vi "2.1 Read Sensor Data.vi"() -> ()   [LabVIEW 2011]
uses:
  <vilib>/Instr/_visa.llb/VISA Configure Serial Port (Instr).vi
panel:
  out "concatenated string":string
  in  "Status":enum16{"Waiting", "Reading", "Time Out!"}(ring)
  in  "stop":bool
  out "Current Status":enum16{"Waiting", "Reading", "Time Out!"}(ring)
  in  "VISA resource name":refnum<visa-resource-name>="COM1"
  in  "error in (no error)":errorcluster
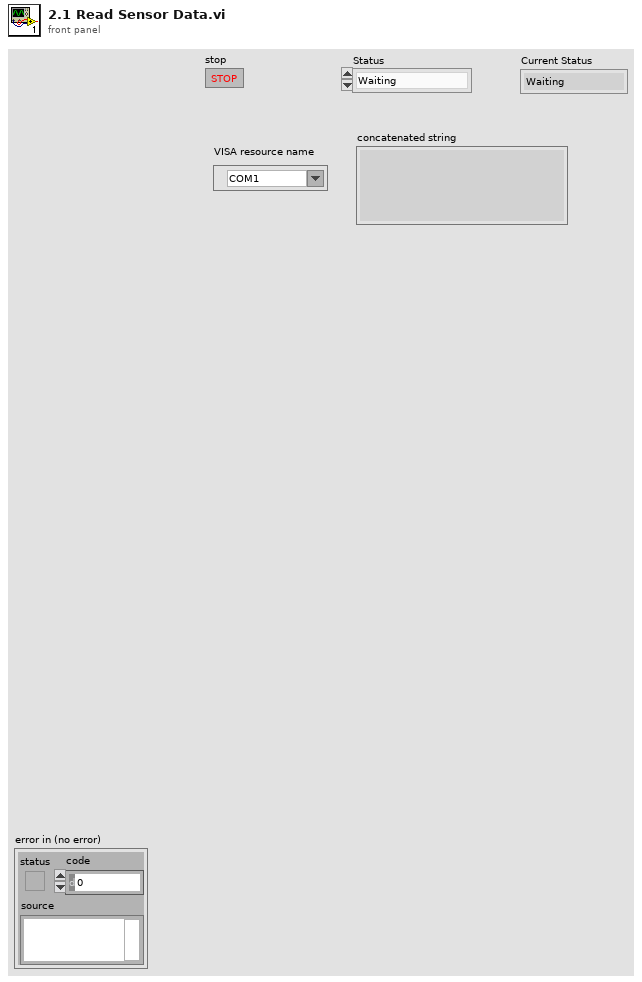
[diagram p1: front panel]
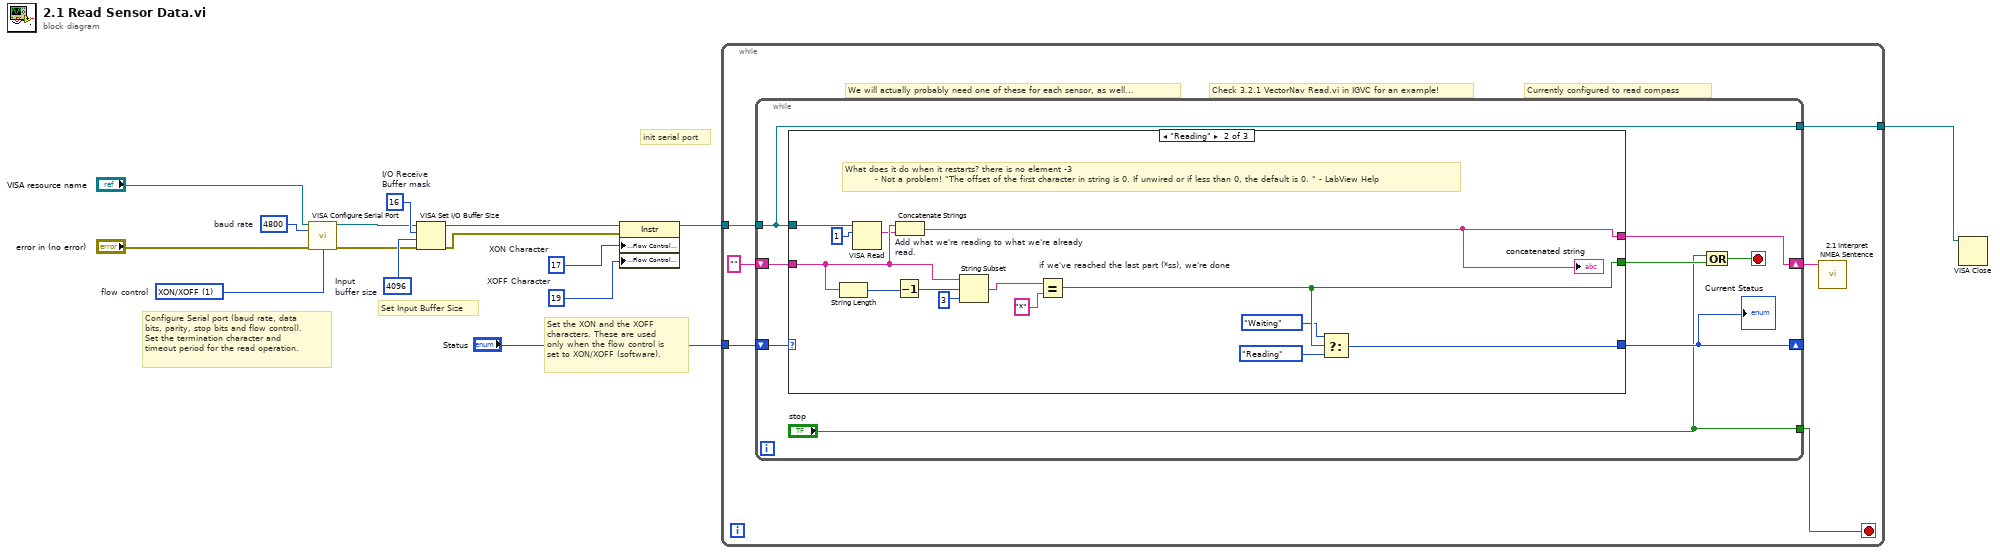
[diagram p0: block diagram]
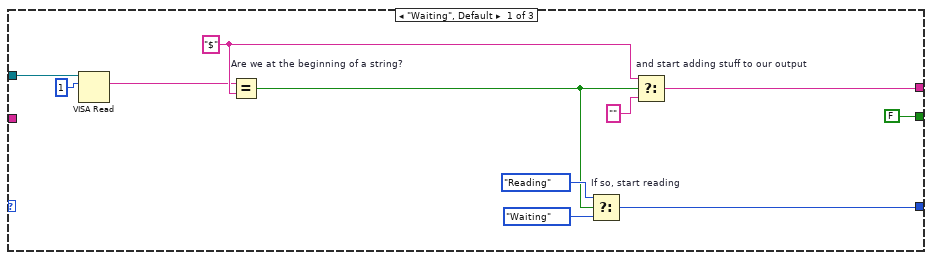
[diagram p2: hidden frame]
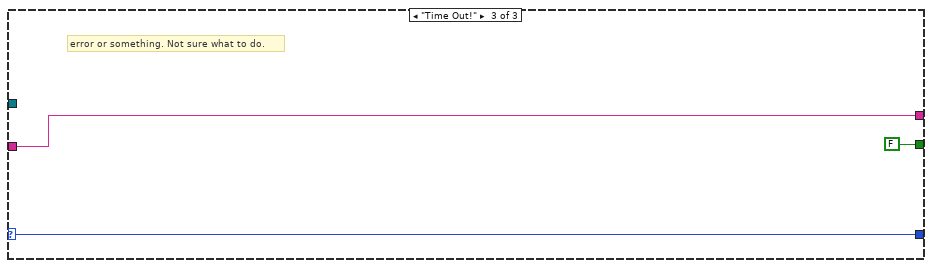
[diagram p3: hidden frame]
diagram:
  w5 = u8 19  # XOFF Character
  w6 = u8 17  # XON Character
  w9 = u32 4096  # Input buffer size
  w10 = u16 16  # I/O Receive Buffer mask
  w12 = u16 1 items=["None"=0, "XON/XOFF"=1, "RTS/CTS"=2, "DTR/DSR"=4]  # flow control
  w14 = u32 4800  # baud rate
  # "Set the XON and the XOFF\ncharacters. These are used\nonly when the flow control is\nset to XON/XOFF (software)."
  # "Set Input Buffer Size"
  # "init serial port"
  # "Configure Serial port (baud rate, data\nbits, parity, stop bits and flow control).\nSet the termination character and\ntimeout period for the read operation."
  n1 = call-poly "VISA Configure Serial Port"("VISA resource name"="VISA resource name", "baud rate (9600)"=w14, "error in (no error)"="error in (no error)", "flow control (0:none)"=w12) -> ("VISA resource name out"=w3:refnum<visa-resource-name>, "error out"=w2:errorcluster)  [unwired: 10 in]
  n2 = VISA Set I/O Buffer Size(VISA resource name=w3, mask (16)=w10, size (4096)=w9, error in (no error)=w2) -> (VISA resource name out=w8:refnum<visa-resource-name>, error out=w7:errorcluster)
  n3 = property class="Instr"(reference=w8, error in=w7, "Serial Settings:Flow Control XON Character"=w6, "Serial Settings:Flow Control XOFF Character"=w5) -> (reference out=w4:refnum<visa-resource-name>)  [unwired: 1 out]
  n4 = while {
    tunnel: "Status" -> [w21]
    tunnel: w4 -> [w18]
    tunnel: [w17] -> w1
    stop <- w16 stop-if-true
    # "Currently configured to read compass"
    # "Check 3.2.1 VectorNav Read.vi in IGVC for an example!"
    # "We will actually probably need one of these for each sensor, as well..."
    n5 = while {
      shift-right: [w28] -> w19
      shift-left: "" -> [w29]
      shift-right: [w25] -> _
      shift-left: w21 -> [w27]
      tunnel: w18 -> [w22]
      tunnel: ["stop"] -> w16
      tunnel: [w22] -> w17
      stop <- w26 stop-if-true
      n6 = case shown="\"Reading\"" w27 {
        selector: w27 -> [_ _ w57]
        tunnel: w29 -> [_ w48 w56]
        tunnel: [w35 w54 w56] -> w28
        tunnel: [w32 w45 w57] -> w25
        tunnel: [FALSE w44 FALSE] -> w24
        tunnel: w22 -> [w31 w42 _]
        frame "Waiting", Default {
          w34 = "$" ("x")
          n7 = VISA Read(VISA resource name=w31, byte count=u32 1) -> (read buffer=w33:string)  [unwired: 1 in, 3 out]
          n8 = Equal? "Are we at the beginning of a string?"(x=w33, y=w34) -> (x = y?=w36:bool)
          n9 = Select "If so, start reading"(t=enum16{"Waiting", "Reading", "Time Out!"}."Reading", s=w36, f=enum16{"Waiting", "Reading", "Time Out!"}."Waiting" ("Current Status")) -> (s? t:f=w32:enum16{"Waiting", "Reading", "Time Out!"})
          n10 = Select "and start adding stuff to our output"(t=w34, s=w36, f="") -> (s? t:f=w35:string)
        }
        frame "Reading" {
          # "What does it do when it restarts? there is no element -3\n          - Not a problem! \"The offset of the first character in string is 0. If unwired or if less than 0, the default is 0. \" - LabView Help"
          n11 = String Length(string=w48) -> (length=w53:i32)
          n12 = VISA Read(VISA resource name=w42, byte count=u32 1) -> (read buffer=w47:string)  [unwired: 1 in, 3 out]
          n13 = Decrement(x=w53) -> (x-1=w52:i32)
          n14 = Concatenate Strings "Add what we're reading to what we're already read."(w48, w47) -> (w54:string)
          "concatenated string" <- w54
          n15 = String Subset(string=w48, offset (0)=w52, length (rest)=3 ("length (rest)")) -> (substring=w50:string)
          n16 = Equal? "if we've reached the last part (*ss), we're done"(x=w50, y="*") -> (x = y?=w44:bool)
          n17 = Select(t=enum16{"Waiting", "Reading", "Time Out!"}."Waiting", s=w44, f=enum16{"Waiting", "Reading", "Time Out!"}."Reading" ("Status")) -> (s? t:f=w45:enum16{"Waiting", "Reading", "Time Out!"})
        }
        frame "Time Out!" {
          # "error or something. Not sure what to do."
        }
      }
      "Current Status" <- w25
      n18 = Compound Arithmetic op=OR("stop", w24) -> (w26:bool)
    }
    n19 = call "2.1 Interpret NMEA Sentence.vi"("NMEA Sentence"=w19) -> ()  [unwired: 11 in]
  }
  n20 = VISA Close(VISA resource name=w1) -> ()  [unwired: 1 in, 1 out]
